vi "Run VI Analyzer.vi"(10 "Number 2":i32, 11 "Number 1":i32) -> (3 "Multiplication":i32)   [LabVIEW 2018]
doc: "This VI is for demonstrating VI Analyzer from CLI and Jenkins"
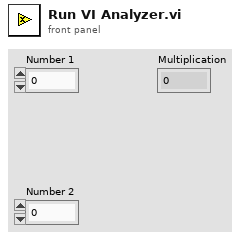
[diagram p1: front panel]
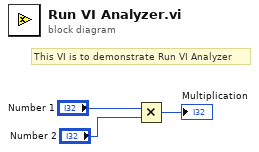
[diagram p0: block diagram]
diagram:
  # "This VI is to demonstrate Run VI Analyzer"
  n1 = Multiply(x="Number 1", y="Number 2") -> (x*y=→"Multiplication":i32)
